vi "System Status Monitor (SubVI).vi"(8 "Refnum in":refnum<k20>) -> (3 "System Status Array":string[](array[string]))   [LabVIEW 2019]
uses:
  <vilib>/ptbypt/NI_PtbyPt.lvlib
  <resource>/objmgr/nicriosae.rc
panel:
  out "Internal Drive Free (MB)":dbl=13807.087616
  # "Time Stamp"
  # "Disk Free GB"
  # "Disk Free %"
  # "Ram Free %"
  # "CPU Utilization %"
  # "Internal HD Free MB"
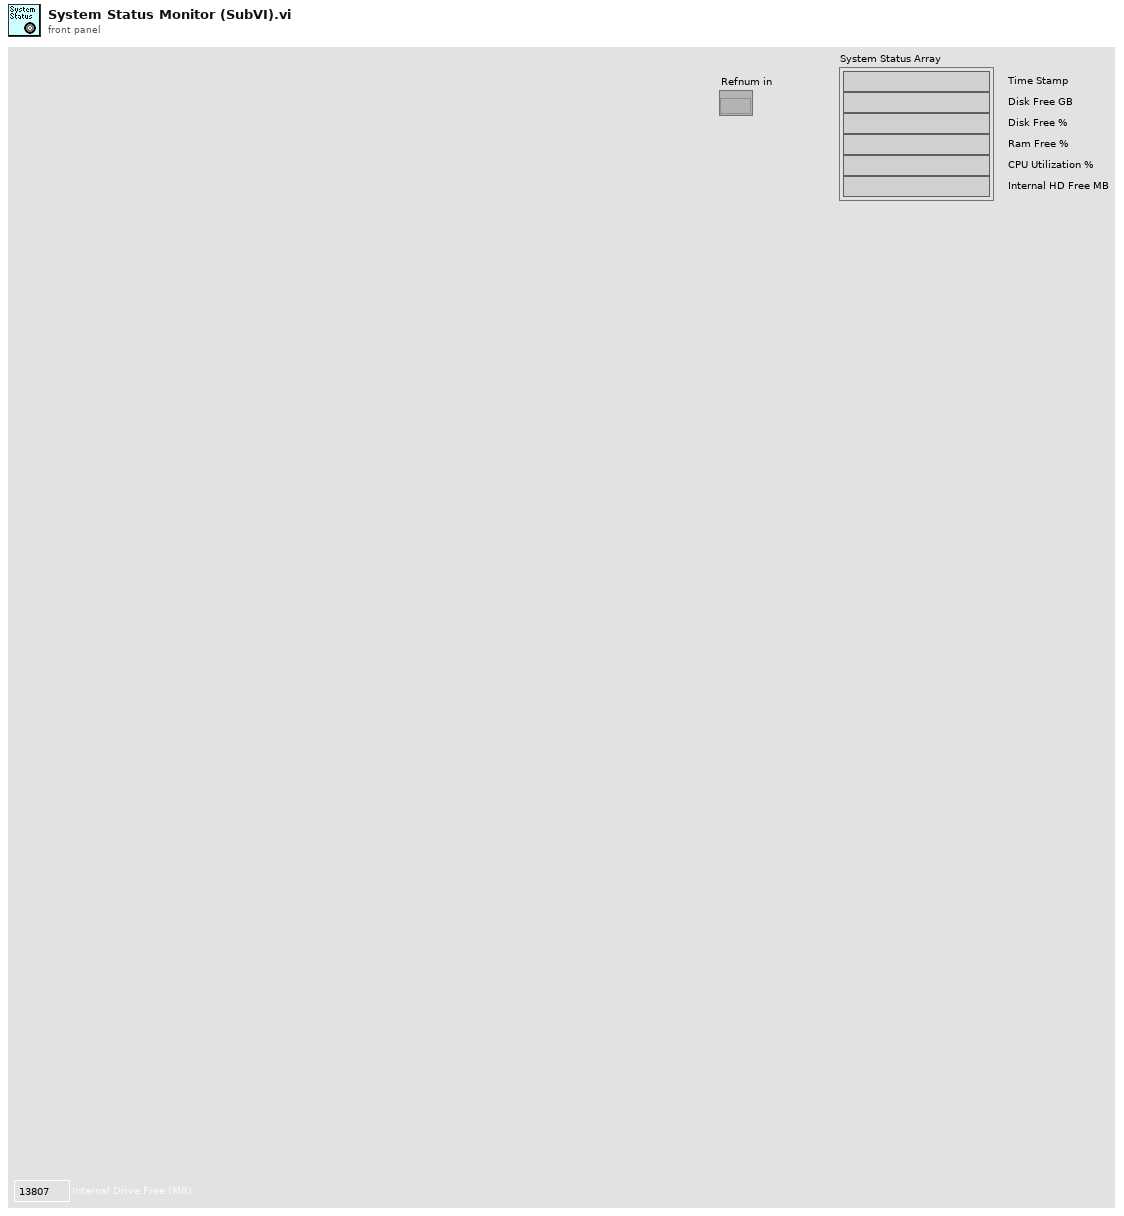
[diagram p1: front panel]
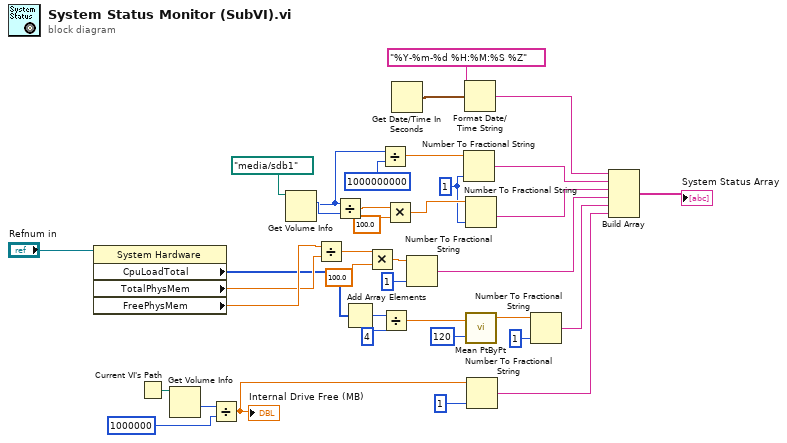
[diagram p0: block diagram]
diagram:
  w14 = i16 1 ("precision (6)")
  n1 = property class="System Hardware"(reference="Refnum in") -> ("CpuLoadTotal"=w21:u32[], "TotalPhysMem"=w32:dbl, "FreePhysMem"=w33:dbl)  [unwired: 1 in, 2 out]
  n2 = Current VI's Path() -> (path=w5:path)
  n3 = Get Volume Info(11:w5) -> (1:w6:i64)  [unwired: 1 in, 5 out]
  n4 = Divide(x=w6, y=i64 1000000) -> (x/y=w3:dbl)
  "Internal Drive Free (MB)" <- w3
  n5 = Get Volume Info(11:path "/media/sdb1" ("file (use dialog)")) -> (1:w7:i64, 2:w8:i64)  [unwired: 1 in, 4 out]
  n6 = Divide(x=w33, y=w32) -> (x/y=w17:dbl)
  n7 = Divide(x=w7, y=w8) -> (x/y=w9:dbl)
  n8 = Add Array Elements(numeric array=w21) -> (sum=w20:u32)
  n9 = Multiply(x=w17, y=100.0) -> (x*y=w36:dbl)
  n10 = Divide(x=w7, y=i64 1000000000) -> (x/y=w25:dbl)
  n11 = Divide(x=w20, y=u32 4 ("x")) -> (x/y=w23:dbl)
  n12 = Multiply(x=w9, y=100.0) -> (x*y=w15:dbl)
  n13 = Get Date/Time In Seconds() -> (seconds since 1Jan1904=w37:timestamp)
  n14 = Number To Fractional String(number=w36, precision (6)=i16 1) -> (F-format string=w29:string)  [unwired: 2 in]
  n15 = Number To Fractional String(number=w25, precision (6)=w14) -> (F-format string=w27:string)  [unwired: 2 in]
  n16 = Format Date/Time String(time format string (%c)="%Y-%m-%d %H:%M:%S %Z", seconds (now)=w37) -> (date/time string=w34:string)  [unwired: 1 in]
  n17 = Number To Fractional String(number=w15, precision (6)=w14) -> (F-format string=w28:string)  [unwired: 2 in]
  n18 = call <vilib>:"Mean PtByPt.vi"("x"=w23, "sample length"=120 ("Samples to average")) -> ("mean"=w24:dbl)  [unwired: 2 in, 1 out]
  n19 = Number To Fractional String(number=w3, precision (6)=i16 1) -> (F-format string=w1:string)  [unwired: 2 in]
  n20 = Number To Fractional String(number=w24, precision (6)=i16 1) -> (F-format string=w30:string)  [unwired: 2 in]
  n21 = Build Array(w34, w27, w28, w29, w30, w1) -> (→"System Status Array":string[])
